vi "Volume img-Init speed chart history.vi"(8 "error in (no error)":errorcluster) -> (0 "error out":errorcluster)   [LabVIEW 2017]
uses:
  Timelapse Viewer/Globals/gl_Time series viewer globals.vi
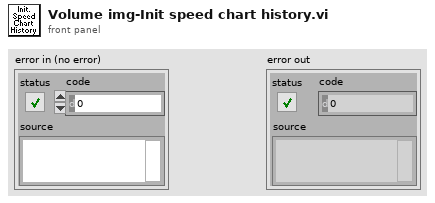
[diagram p1: front panel]
types:
  T1 = typedef "AVI playback header info cluster.ctl" = cluster{"Frame Size":u32, "AOD fill time (us)":dbl, "Dwell time (us)":dbl, "Frame period (ms)":dbl, "Number of Miniscans":u16, "Number of Pixels in Miniscan":u16}
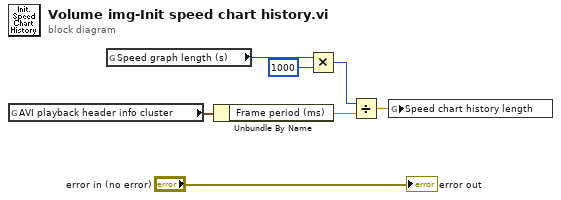
[diagram p0: block diagram]
diagram:
  n1 = global read "gl_Time series viewer globals.vi" "AVI playback header info cluster"() -> (w3:T1)
  n2 = global read "gl_Time series viewer globals.vi" "Speed graph length (s)"() -> (w1:i32)
  n3 = Unbundle By Name(w3) -> ("Frame period (ms)"=w4:dbl)
  n4 = Multiply(x=w1, y=1000) -> (x*y=w7:i32)
  n5 = Divide(x=w7, y=w4) -> (x/y=w5:dbl)
  n6 = global write "gl_Time series viewer globals.vi" "Speed chart history length"(w5) -> ()
  "error out" <- "error in (no error)"
